vi "CantLayerGen.vi"(6 "Layer":u32=160, 9 "OHpows":dbl[](array[numeric]), 10 "HatchPow":T6={"Power"=300.0, "Mark Speed"=400.0, "Jump Speed"=1000.0}, 11 "RectHatch":T7={"Width"=10.0, "Height"=10.0, "Angle"=45.0, "OffX"=0.1, "OffY"=0.1, "Spacing"=0.1} {"Spacing" format="%#_13g"; "OffY" format="%#_13g"; "OffX" format="%#_13g"; "Height" format="%#_13g"; "Width" format="%#_13g"}) -> (1 "Hatches2":T1(array[cluster]), 2 "Hatches":T1(array[cluster]), 3 "PathSups":T2[](array[typedef]))   [LabVIEW 2014]
uses:
  TypeDefs/RectHatch.ctl
  TypeDefs/PowerSpeed.ctl
  TypeDefs/PathSupreme.ctl
  PSup2SCAN/Sub/VelocityProfile.ctl
  PSup2SCAN/Sub/PathCut.ctl
  PSup2SCAN/Sub/Segment.ctl
  PSup2SCAN/Sub/Point.ctl
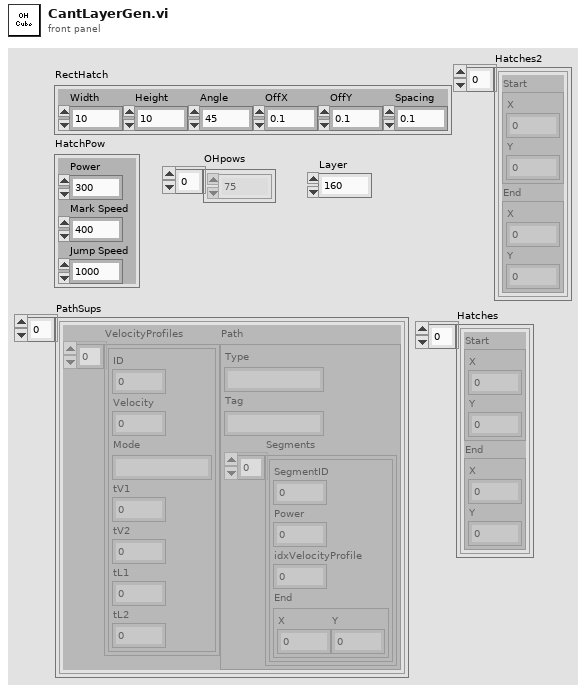
[diagram p1: front panel]
types:
  T1 = cluster{"Start":cluster{"X":dbl, "Y":dbl}, "End":cluster{"X":dbl, "Y":dbl}}[]
  T2 = typedef "PathSupreme.ctl" = cluster{"VelocityProfiles":T3[], "Path":T4}
  T3 = typedef "VelocityProfile.ctl" = cluster{"ID":u32, "Velocity":dbl, "Mode":string, "tV1":u32, "tV2":u32, "tL1":u32, "tL2":u32}
  T4 = typedef "PathCut.ctl" = cluster{"Type":string, "Tag":string, "Segments":T5[]}
  T5 = typedef "Segment.ctl" = cluster{"SegmentID":u16, "Power":sgl, "idxVelocityProfile":u16, "End":cluster{"X":sgl, "Y":sgl}}
  T6 = typedef "PowerSpeed.ctl" = cluster{"Power":dbl, "Mark Speed":dbl, "Jump Speed":dbl}
  T7 = typedef "RectHatch.ctl" = cluster{"Width":dbl, "Height":dbl, "Angle":sgl, "OffX":dbl, "OffY":dbl, "Spacing":dbl}
  T8 = typedef "Point.ctl" = cluster{"X":dbl, "Y":dbl}
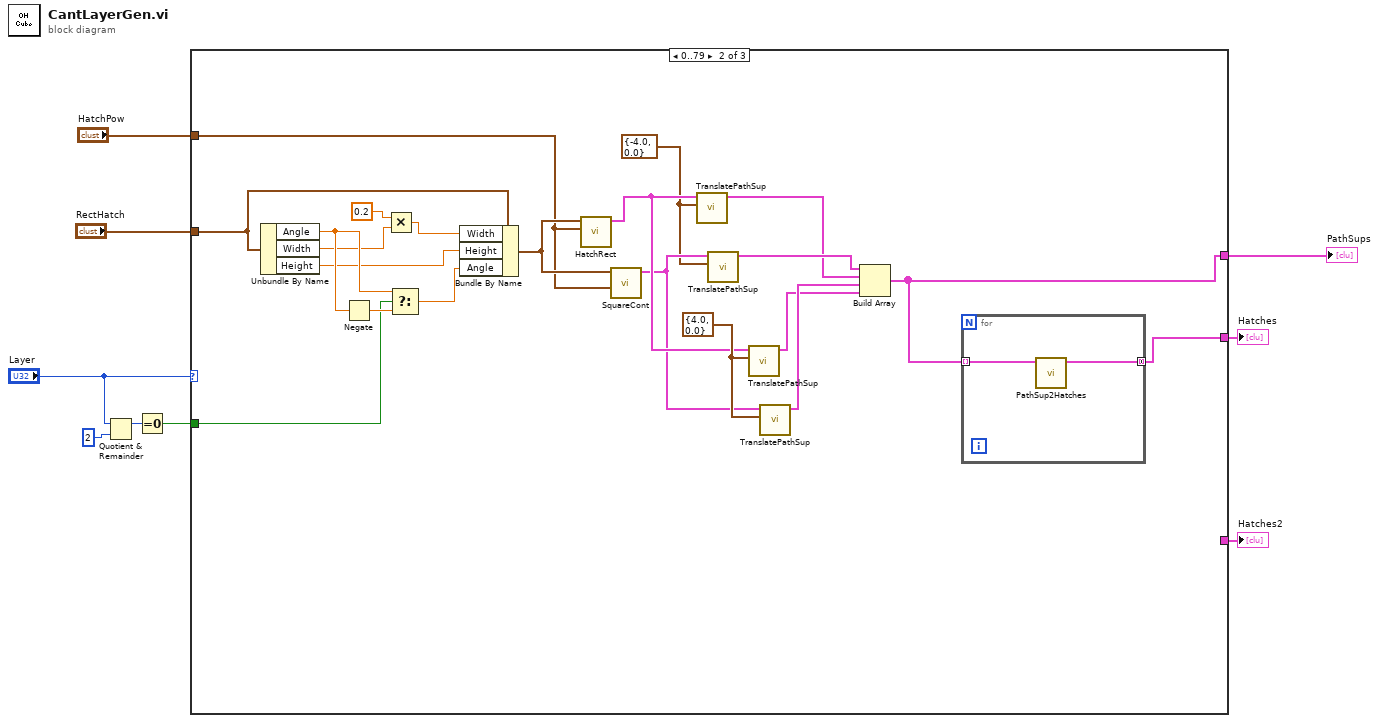
[diagram p0: block diagram]
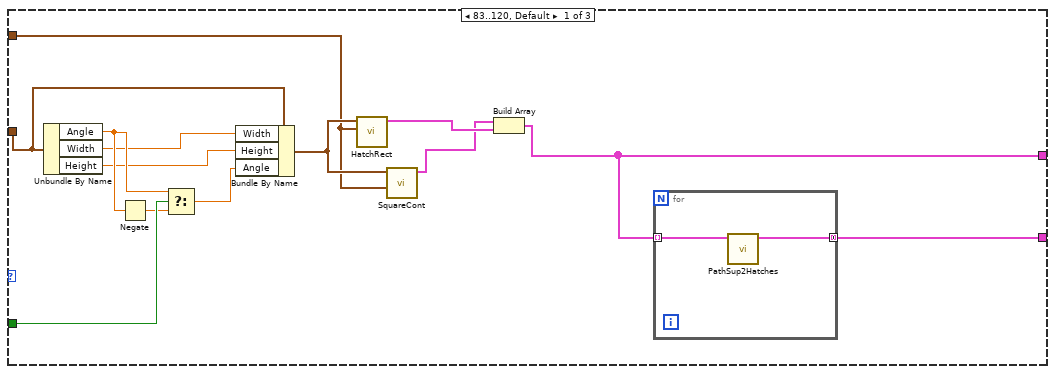
[diagram p2: hidden frame]
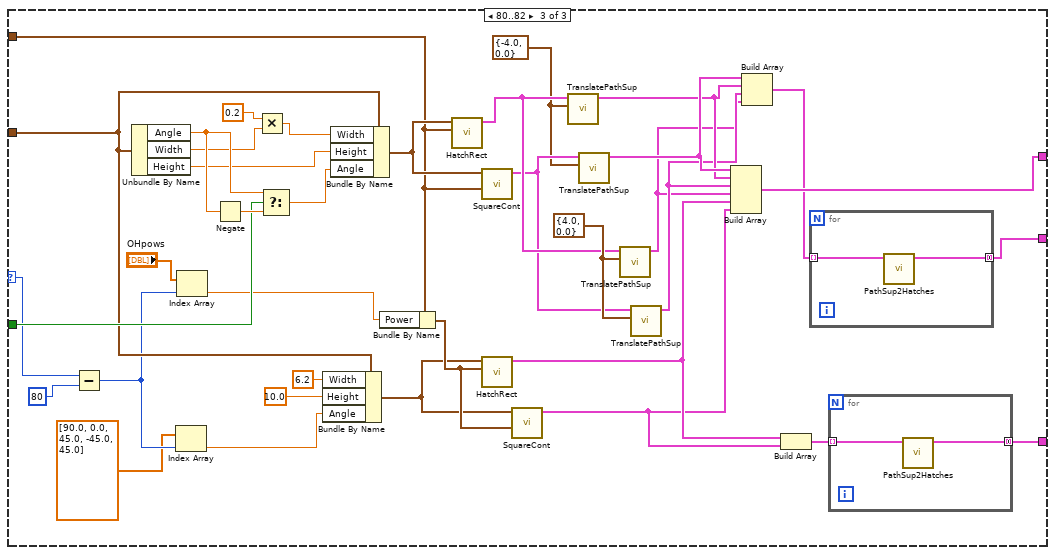
[diagram p3: hidden frame]
diagram:
  n1 = Quotient & Remainder(x="Layer", y=u8 2) -> (x-y*floor(x/y)=w9:u32)  [unwired: 1 out]
  n2 = Equal To 0?(x=w9) -> (x = 0?=w6:bool)
  n3 = case shown="0..79" "Layer" {
    selector: "Layer" -> [_ _ w61]
    tunnel: w6 -> [w22 w40 w72]
    tunnel: "RectHatch" -> [w21 w39 w69]
    tunnel: "HatchPow" -> [w16 w41 w71]
    tunnel: [w11 w26 w65] -> w3
    tunnel: [w10 w25 w52] -> w2
    tunnel: [_ _ w48] -> w1
    frame 83..120, Default {
      n4 = Unbundle By Name(w21) -> ("Angle"=w19:sgl, "Width"=w15:dbl, "Height"=w14:dbl)
      n5 = Negate(x=w19) -> (-x=w20:sgl)
      n6 = Select(t=w19, s=w22, f=w20) -> (s? t:f=w18:sgl)
      n7 = Bundle By Name(cluster=w21, "Width"=w15, "Height"=w14, "Angle"=w18) -> (w17:T7)
      n8 = call "HatchRect.vi"("HatchPow"=w16, "RectHatch"=w17) -> ("PathSupreme"=w13:T2)  [unwired: 9 in]
      n9 = call "SquareCont.vi"("ContPow"=w16, "RectHatch"=w17) -> ("PathSupreme"=w12:T2)  [unwired: 9 in]
      n10 = Build Array(w12, w13) -> (w11:T2[])
      n11 = for {
        tunnel: w11 -> [w24] mode=indexing
        tunnel: [w23] -> w10 mode=concatenating
        n12 = call "PathSup2Hatches.vi"("PathSupOut"=w24) -> ("Hatches"=w23:T1)  [unwired: 10 in]
      }
    }
    frame 0..79 {
      w31 = T8 {"X"=-4.0, "Y"=0.0} ("Offset")
      w38 = T8 {"X"=4.0, "Y"=0.0} ("Offset")
      n13 = Unbundle By Name(w39) -> ("Angle"=w44:sgl, "Width"=w33:dbl, "Height"=w35:dbl)
      n14 = Negate(x=w44) -> (-x=w45:sgl)
      n15 = Multiply(x=0.2 ("Width"), y=w33) -> (x*y=w32:dbl)
      n16 = Select(t=w44, s=w40, f=w45) -> (s? t:f=w43:sgl)
      n17 = Bundle By Name(cluster=w39, "Width"=w32, "Height"=w35, "Angle"=w43) -> (w42:T7)
      n18 = call "HatchRect.vi"("HatchPow"=w41, "RectHatch"=w42) -> ("PathSupreme"=w37:T2)  [unwired: 9 in]
      n19 = call "SquareCont.vi"("ContPow"=w41, "RectHatch"=w42) -> ("PathSupreme"=w36:T2)  [unwired: 9 in]
      n20 = call "TranslatePathSup.vi"("Offset"=w31, "PathSupreme"=w37) -> ("PathSupOut"=w29:T2)  [unwired: 9 in]
      n21 = call "TranslatePathSup.vi"("Offset"=w31, "PathSupreme"=w36) -> ("PathSupOut"=w30:T2)  [unwired: 9 in]
      n22 = call "TranslatePathSup.vi"("Offset"=w38, "PathSupreme"=w37) -> ("PathSupOut"=w27:T2)  [unwired: 9 in]
      n23 = call "TranslatePathSup.vi"("Offset"=w38, "PathSupreme"=w36) -> ("PathSupOut"=w28:T2)  [unwired: 9 in]
      n24 = Build Array(w30, w29, w28, w27) -> (w26:T2[])
      n25 = for {
        tunnel: w26 -> [w47] mode=indexing
        tunnel: [w46] -> w25 mode=concatenating
        n26 = call "PathSup2Hatches.vi"("PathSupOut"=w47) -> ("Hatches"=w46:T1)  [unwired: 10 in]
      }
    }
    frame 80..82 {
      w73 = T8 {"X"=-4.0, "Y"=0.0} ("Offset")
      w80 = T8 {"X"=4.0, "Y"=0.0} ("Offset")
      n27 = Subtract(x=w61, y=u32 80) -> (x-y=w60:u32)
      n28 = Unbundle By Name(w69) -> ("Angle"=w83:sgl, "Width"=w75:dbl, "Height"=w77:dbl)
      n29 = Index Array(array=dbl[] [90.0, 0.0, 45.0, -45.0, 45.0], index=w60) -> (element=w58:dbl)
      n30 = Index Array(array="OHpows", index=w60) -> (element=w63:dbl)
      n31 = Negate(x=w83) -> (-x=w84:sgl)
      n32 = Multiply(x=0.2 ("Width"), y=w75) -> (x*y=w74:dbl)
      n33 = Select(t=w83, s=w72, f=w84) -> (s? t:f=w82:sgl)
      n34 = Bundle By Name(cluster=w69, "Width"=6.2, "Height"=10.0, "Angle"=w58) -> (w66:T7)
      n35 = Bundle By Name(cluster=w69, "Width"=w74, "Height"=w77, "Angle"=w82) -> (w81:T7)
      n36 = Bundle By Name(cluster=w71, "Power"=w63) -> (w70:T6)
      n37 = call "HatchRect.vi"("HatchPow"=w71, "RectHatch"=w81) -> ("PathSupreme"=w79:T2)  [unwired: 9 in]
      n38 = call "SquareCont.vi"("ContPow"=w71, "RectHatch"=w81) -> ("PathSupreme"=w78:T2)  [unwired: 9 in]
      n39 = call "HatchRect.vi"("HatchPow"=w70, "RectHatch"=w66) -> ("PathSupreme"=w51:T2)  [unwired: 9 in]
      n40 = call "SquareCont.vi"("ContPow"=w70, "RectHatch"=w66) -> ("PathSupreme"=w50:T2)  [unwired: 9 in]
      n41 = call "TranslatePathSup.vi"("Offset"=w73, "PathSupreme"=w79) -> ("PathSupOut"=w56:T2)  [unwired: 9 in]
      n42 = call "TranslatePathSup.vi"("Offset"=w73, "PathSupreme"=w78) -> ("PathSupOut"=w57:T2)  [unwired: 9 in]
      n43 = call "TranslatePathSup.vi"("Offset"=w80, "PathSupreme"=w79) -> ("PathSupOut"=w54:T2)  [unwired: 9 in]
      n44 = call "TranslatePathSup.vi"("Offset"=w80, "PathSupreme"=w78) -> ("PathSupOut"=w55:T2)  [unwired: 9 in]
      n45 = Build Array(w57, w56, w55, w54, w51, w50) -> (w65:T2[])
      n46 = Build Array(w57, w56, w55, w54) -> (w53:T2[])
      n47 = Build Array(w51, w50) -> (w49:T2[])
      n48 = for {
        tunnel: w53 -> [w88] mode=indexing
        tunnel: [w87] -> w52 mode=concatenating
        n49 = call "PathSup2Hatches.vi"("PathSupOut"=w88) -> ("Hatches"=w87:T1)  [unwired: 10 in]
      }
      n50 = for {
        tunnel: w49 -> [w86] mode=indexing
        tunnel: [w85] -> w48 mode=concatenating
        n51 = call "PathSup2Hatches.vi"("PathSupOut"=w86) -> ("Hatches"=w85:T1)  [unwired: 10 in]
      }
    }
  }
  "PathSups" <- w3
  "Hatches" <- w2
  "Hatches2" <- w1
